vi "PV Initialize.vi"(6 "Timeout Value":u32=1000 min=30 max=2000 step=1, 8 "error in (no error)":errorcluster, 11 "VISA session in":refnum<visa-resource-name>) -> (0 "error out":errorcluster {"code" format="%.0x"}, 3 "VISA session out":refnum<visa-resource-name>)   [LabVIEW 2018, in "Pfeiffer Vacuum.lvlib"]
doc: "This VI passes the addressing information in the instrument descriptor to the Instr Open VI. You must run this VI before using any of the instrument driver VIs for this instrument. \n\nWARNINGS: \n(1) You MUSThave VISA Version 2.0 or higher installed to use this Instrument driver. \n(2) For RS 232 only"
uses:
  Pfeiffer Vacuum.lvlib
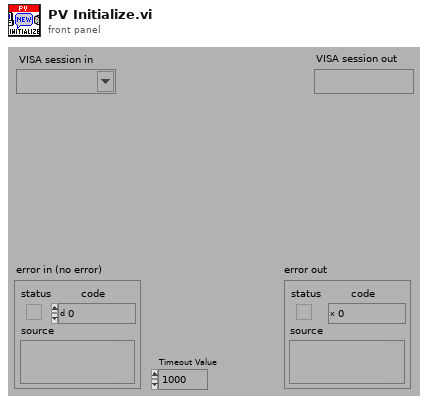
[diagram p1: front panel]
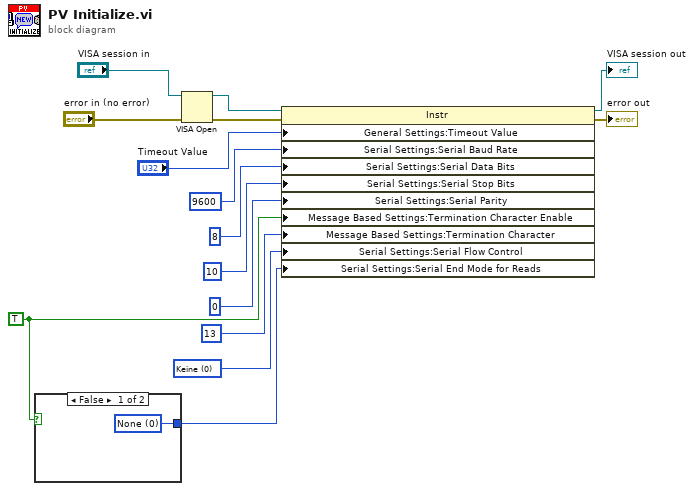
[diagram p0: block diagram]
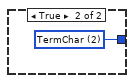
[diagram p2: hidden frame]
diagram:
  w8 = TRUE
  w10 = u16 0 items=["Keine", "XON/XOFF", "RTS/CTS", "XON/XOFF & RTS/CTS", "DTR/DSR", "XON/XOFF & DTR/DSR"] ("flow control (0:none)")
  n1 = case shown="False" w8 {
    tunnel: [w16 w17] -> w15
    frame False {
      w16 = u16 0 items=["None", "LastBit", "TermChar"] ("Serial Settings:Serial End Mode for Reads")
    }
    frame True {
      w17 = u16 2 items=["None", "LastBit", "TermChar"] ("Serial Settings:Serial End Mode for Reads")
    }
  }
  n2 = VISA Open(error in (no error)="error in (no error)", VISA resource name="VISA session in") -> (VISA resource name=w4:refnum<visa-resource-name>, error out=w2:errorcluster)  [unwired: 3 in]
  n3 = property class="Instr"(reference=w4, error in=w2, "General Settings:Timeout Value"="Timeout Value", "Serial Settings:Serial Baud Rate"=u32 9600, "Serial Settings:Serial Data Bits"=u16 8 ("ASRL Parity"), "Serial Settings:Serial Stop Bits"=u16 10 ("ASRL Stop Bits"), "Serial Settings:Serial Parity"=u16 0 ("ASRL Data Bits"), "Message Based Settings:Termination Character Enable"=w8, "Message Based Settings:Termination Character"=u8 13 ("termination char\n(0xA = '\\n' = LF)"), "Serial Settings:Serial Flow Control"=w10, "Serial Settings:Serial End Mode for Reads"=w15) -> (reference out=→"VISA session out":refnum<visa-resource-name>, error out=→"error out":errorcluster)
